vi "24-Host Accepts On-Line Request from Equipment.vi"(8 "error in":errorcluster) -> (0 "error out":errorcluster, 2 "Timeout":bool, 3 "On-Line":bool)   [LabVIEW 2020, in "SECS Scenarios.lvlib" / "Scenarios Class.lvclass"]
uses:
  Scenarios Class.lvclass
  24-Host Accepts On-Line Request from Equipment.ctl
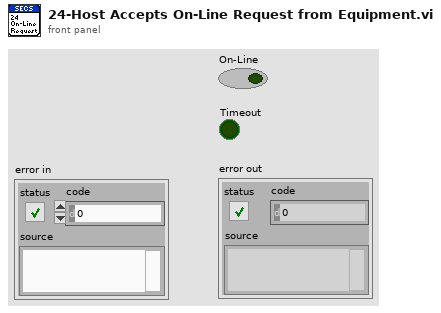
[diagram p1: front panel]
types:
  T1 = typedef "SECS Scenarios.lvlib/Scenarios Class.lvclass/24-Host Accepts On-Line Request from Equipment.ctl" = cluster{"Reply Notifier":refnum<notifier>}
  T2 = typedef "SECS Scenarios.lvlib/Scenarios Class.lvclass/Request Refnum.ctl" = cluster{"11-Alarm Management":refnum<user-event>, "07-Event Report From Equipment":refnum<user-event>, "14-Process Program Creating Editing or Deleting":refnum<user-event>, "21-Material Movement":refnum<user-event>, "23-Equipment Sends Information to Host":refnum<user-event>, "24-Host Accepts On-Line Request from Equipment":refnum<user-event>, "25-Host Refuses On-Line Request":refnum<user-event>, "29-Equipment Requests Time Value from Host":refnum<user-event>, "33-Update Trace Data":refnum<user-event>}
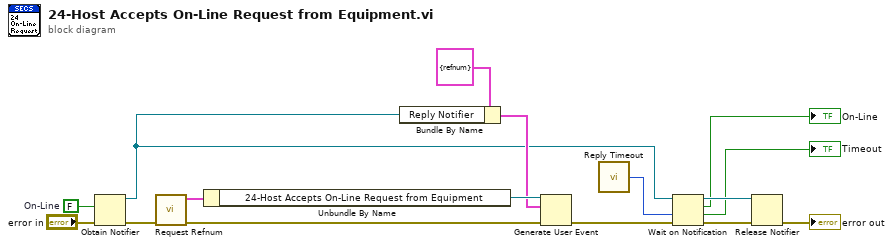
[diagram p0: block diagram]
diagram:
  w9 = FALSE  # On-Line
  n1 = Obtain Notifier(notification data type=w9, error in (no error)="error in") -> (notifier out=w4:refnum<notifier>, error out=w10:errorcluster)  [unwired: 2 in, 1 out]
  n2 = call "Request Refnum.vi"("error in"=w10) -> ("error out"=w15:errorcluster, "Request Refnum"=w16:T2)  [unwired: 9 in]
  n3 = Unbundle By Name(w16) -> ("24-Host Accepts On-Line Request from Equipment"=w14:refnum<user-event>)
  n4 = Bundle By Name(cluster=T1 {"Reply Notifier"=refnum} ("24-Host Accepts On-Line Request from Equipment"), "Reply Notifier"=w4) -> (w13:T1)
  n5 = Generate User Event(user event=w14, event data cluster=w13, error in=w15) -> (error out=w5:errorcluster)  [unwired: 1 in, 1 out]
  n6 = call "Reply Timeout.vi"() -> ("Reply Timeout"=w8:i32)
  n7 = Wait on Notification(notifier=w4, timeout in ms (-1)=w8, error in (no error)=w5) -> (notifier out=w7:refnum<notifier>, notification=→"On-Line":bool, timed out?=→"Timeout":bool, error out=w6:errorcluster)  [unwired: 1 in]
  n8 = Release Notifier(notifier=w7, error in (no error)=w6) -> (error out=→"error out":errorcluster)  [unwired: 1 in, 2 out]
